vi "Change Delimiters.vi"(8 "Error In":errorcluster, 11 "Lexer In":refnum<class "Lexer.lvclass">) -> (0 "Error Out":errorcluster, 3 "Lexer Out":refnum<class "Lexer.lvclass">)   [LabVIEW 2018, in "Toolkit.lvlib" / "Lexer.lvclass"]
uses:
  Lexer.lvclass
  Lexer.lvclass/Lexer.ctl
  Type Definitions/Delimiters.ctl
  Tokens/SetDelimiter/SetDelimiter.lvclass
  D:/Users/cfield/Code/Field R&D Services/Mustache/LabVIEW/trunk/src/Toolkit/Low-Level/Tokens/Abstract/Abstract.lvclass
  Toolkit.lvlib
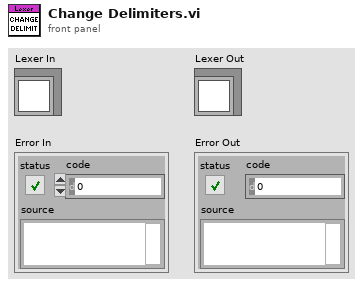
[diagram p1: front panel]
types:
  T1 = typedef "Toolkit.lvlib/Delimiters.ctl" = cluster{"Close":string, "Open":string}
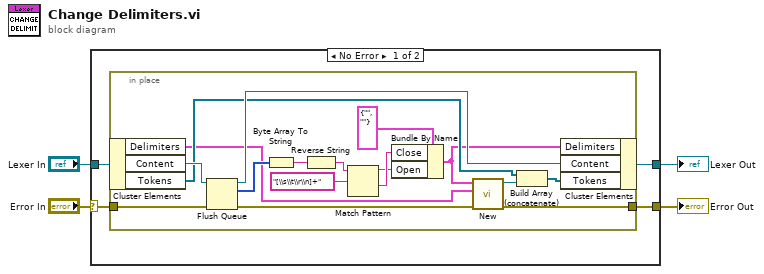
[diagram p0: block diagram]
diagram:
  n1 = case shown="No Error" "Error In" {
    selector: "Error In" -> [w5 w26]
    tunnel: [w8 w26] -> w4
    tunnel: [w7 w27] -> w3
    tunnel: "Lexer In" -> [w6 w27]
    frame No Error {
      n2 = in-place {
        in-place-border: [w14] -> w8
        in-place-border: w5 -> [w19]
        n3 = in-place-cluster #1(w6) -> ("Delimiters"=w9:T1, "Content"=w25:refnum<queue>, "Tokens"=w18:refnum<class "Abstract.lvclass">[])
        n4 = Flush Queue(queue=w25, error in (no error)=w19) -> (queue out=w22:refnum<queue>, remaining elements=w24:u8[], error out=w15:errorcluster)
        n5 = Byte Array To String(unsigned byte array=w24) -> (string=w23:string)
        n6 = Reverse String(1:w23) -> (0:w21:string)
        n7 = Match Pattern(string=w21, regular expression="[\\s\\t\\r\\n]+") -> (before substring=w12:string, after substring=w13:string)  [unwired: 1 in, 2 out]
        n8 = Bundle By Name(cluster=T1 {"Close"="", "Open"=""} ("Delimiters"), "Close"=w13, "Open"=w12) -> (w10:T1)
        n9 = call "New.vi"("Error In"=w15, "Old Delimiters"=w9, "New Delimiters"=w10) -> ("Error Out"=w14:errorcluster, "SetDelimiter"=w17:refnum<class "SetDelimiter.lvclass">)  [unwired: 7 in]
        n10 = Build Array (concatenate)(w18, w17) -> (w16:refnum<class "Abstract.lvclass">[])
        n11 = in-place-cluster #1("Delimiters"=w10, "Content"=w22, "Tokens"=w16) -> (w7:refnum<class "Lexer.lvclass">)
      }
    }
    frame Error {
    }
  }
  "Error Out" <- w4
  "Lexer Out" <- w3
